vi "Read Parent.vi"(8 "error in (no error)":errorcluster, 11 "Asset Location in":refnum<class "Asset Location.lvclass">) -> (0 "error out":errorcluster, 2 "parent":string, 3 "Asset Location out":refnum<class "Asset Location.lvclass">)   [LabVIEW 2019, in "Asset Location.lvclass"]
uses:
  Asset Location.lvclass
  Asset Location.lvclass/Asset Location.ctl
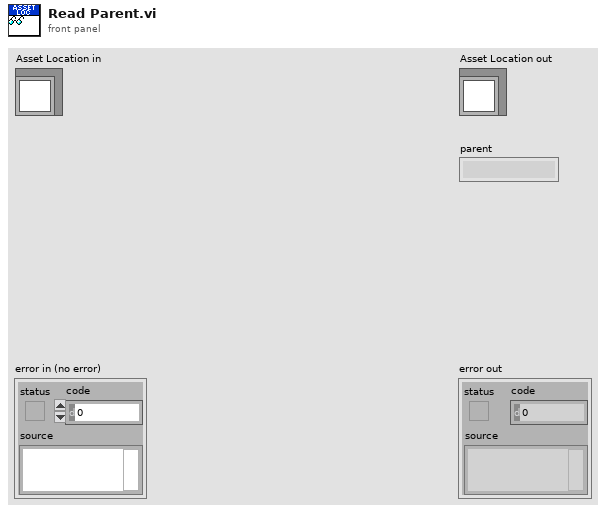
[diagram p1: front panel]
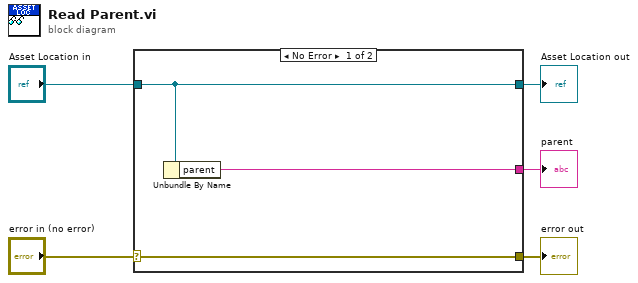
[diagram p0: block diagram]
diagram:
  n1 = case shown="No Error" "error in (no error)" {
    selector: "error in (no error)" -> [w8 w9]
    tunnel: [w8 w9] -> w4
    tunnel: [w7 w10] -> w2
    tunnel: "Asset Location in" -> [w7 w10]
    tunnel: [w6 _] -> w1
    frame No Error {
      n2 = Unbundle By Name(w7) -> ("parent"=w6:string)
    }
    frame Error {
    }
  }
  "error out" <- w4
  "Asset Location out" <- w2
  "parent" <- w1
